vi "4-20mA Settings.vi"(8 "error in (no error)":errorcluster, 11 "PRM Config In":T1={"GUID"="", "Drop Coords"={"Horizontal"=0, "Vertical"=0}, "Process Name"="", "Settings"={"Cycle Period"=500.0, "PID 2 Parameters"={"Input Device"=enum."Default", "Output Device"=enum."Default", "Setpoint"=0.0, "PID gains"={"proportional gain (Kc)"=1.0, "integral time (Ti, min)"=0.01, "derivative time (Td, min)"=0.0}, "output range"={"output low"=0.02, "output high"=0.0}}, "Manual Entry"=0.0, "Auto?"=TRUE, "4-20mA Input Settings"={"Input Channel "=0}, "4-20mA Out Settings"={"Output DAQ Task"=""}, "Input Channel Tag Name "=""}, "Settings Load Count"=0} {"Settings"."PID 2 Parameters"."output range"."output low" format="%.2f"; "Settings"."PID 2 Parameters"."output range"."output high" min=0.0 max=100.0 format="%.2f"; "Settings"."PID 2 Parameters"."PID gains"."derivative time (Td, min)" format="%.3f"; "Settings"."PID 2 Parameters"."PID gains"."integral time (Ti, min)" format="%.3f"; "Settings"."PID 2 Parameters"."PID gains"."proportional gain (Kc)" format="%.3f"}) -> (0 "error out":errorcluster, 3 "PRM Config Out":T1={"GUID"="", "Drop Coords"={"Horizontal"=0, "Vertical"=0}, "Process Name"="", "Settings"={"Cycle Period"=500.0, "PID 2 Parameters"={"Input Device"=enum."Default", "Output Device"=enum."Default", "Setpoint"=0.0, "PID gains"={"proportional gain (Kc)"=1.0, "integral time (Ti, min)"=0.01, "derivative time (Td, min)"=0.0}, "output range"={"output low"=0.02, "output high"=0.0}}, "Manual Entry"=0.0, "Auto?"=TRUE, "4-20mA Input Settings"={"Input Channel "=0}, "4-20mA Out Settings"={"Output DAQ Task"=""}, "Input Channel Tag Name "=""}, "Settings Load Count"=0} {"Settings"."PID 2 Parameters"."output range"."output low" format="%.2f"; "Settings"."PID 2 Parameters"."output range"."output high" min=0.0 max=100.0 format="%.2f"; "Settings"."PID 2 Parameters"."PID gains"."derivative time (Td, min)" format="%.3f"; "Settings"."PID 2 Parameters"."PID gains"."integral time (Ti, min)" format="%.3f"; "Settings"."PID 2 Parameters"."PID gains"."proportional gain (Kc)" format="%.3f"})   [LabVIEW 2018, in "4-20mA Module.lvlib"]
uses:
  4-20mA Module.lvlib
  KNF Pump/Settings Cluster plus SIMDOS.ctl
  KNF Pump/KNF SIMDOS.lvlib
  Ismatec ISM 831C/Ismatec ISM 831C.lvlib
  VICI M50 Party Mode/VICI M6 M50 Party Mode.lvlib
  Masterflex 7550-30/Masterflex 7550-30.lvlib
  Mettler Toledo/Mettler Toledo.lvlib
  Bronkhorst M13 Flow Meter/Bronkhorst M13 Flow Meter.lvlib
  Bronkhorst M14 Flow Meter/Bronkhorst M14 Flow Meter.lvlib
  Settings/Settings.lvlib
  <vilib>/Utility/xml.llb/Write to XML File(string).vi
  <vilib>/Utility/miscctls.llb/LVPoint32TypeDef.ctl
  Masterflex 7550-30/Controls/Settings Cluster.ctl
  Mettler Toledo/Controls/Settings Cluster.ctl
  Bronkhorst M13 Flow Meter/Settings Cluster.ctl
  Measure Instrument/PID Input Enum.ctl
  Measure Instrument/PID 2 Output Enum.ctl
  Controls/Pressure Regulator COM Settings.ctl
  Pressure Transmitter/Pressure Transmitter Device Settings.ctl
  Pressure Transmitter/Pressure Transmitter Library.lvlib
  Controls/4-20mA Module Settings Cluster.ctl
  Controls/4-20mA Module Config Cluster.ctl
  Pressure Reg Module/Pressure Regulator Device Settings.ctl
  Pressure Reg Module/Pressure Regulator Library.lvlib
panel:
  out "Cancelled?":bool=TRUE
  in  "Cancel Button":bool
  in  "OK Button":bool
  in  "Settings Dialog":T12={"Cycle Period"=500.0, "Masterflex"={"VISA resource name"="", "Simulated?"=FALSE, "Pump Number"=1.0, "Reverse?"=FALSE}, "Mettler"={"VISA resource name"="", "Simulated?"=FALSE}, "Bronkhorst M13 Flow Meter"={"VISA resource name"="", "Simulated?"=FALSE}, "PID Parameters"={"Input Device"=enum."Default", "Output Device"=enum."Default", "PID gains"={"proportional gain (Kc)"=1.0, "integral time (Ti, min)"=0.01, "derivative time (Td, min)"=0.0}}, "PID Range"={"output high"=100.0, "output low"=0.0}, "Pressure Regulator Settings"={"Analog DAQ Task"="", "Digital DAQ Task"="", "Value"=0.02, "On?"=FALSE}} {"Pressure Regulator Settings"."Value" min=0.004 max=0.02; "PID Range"."output low" min=0.0 max=100.0 format="%.2f"; "PID Range"."output high" format="%.2f"; "PID Parameters"."PID gains"."derivative time (Td, min)" format="%.3f"; "PID Parameters"."PID gains"."integral time (Ti, min)" format="%.3f"; "PID Parameters"."PID gains"."proportional gain (Kc)" format="%.3f"; "Masterflex"."Pump Number" min=1.0 max=20.0 step=1.0}
  out "UI Refresh Needed?":bool
  # "Instrument Settings"
  # "Instrument Settings"
  # "Instrument Settings"
  # "Instrument Settings"
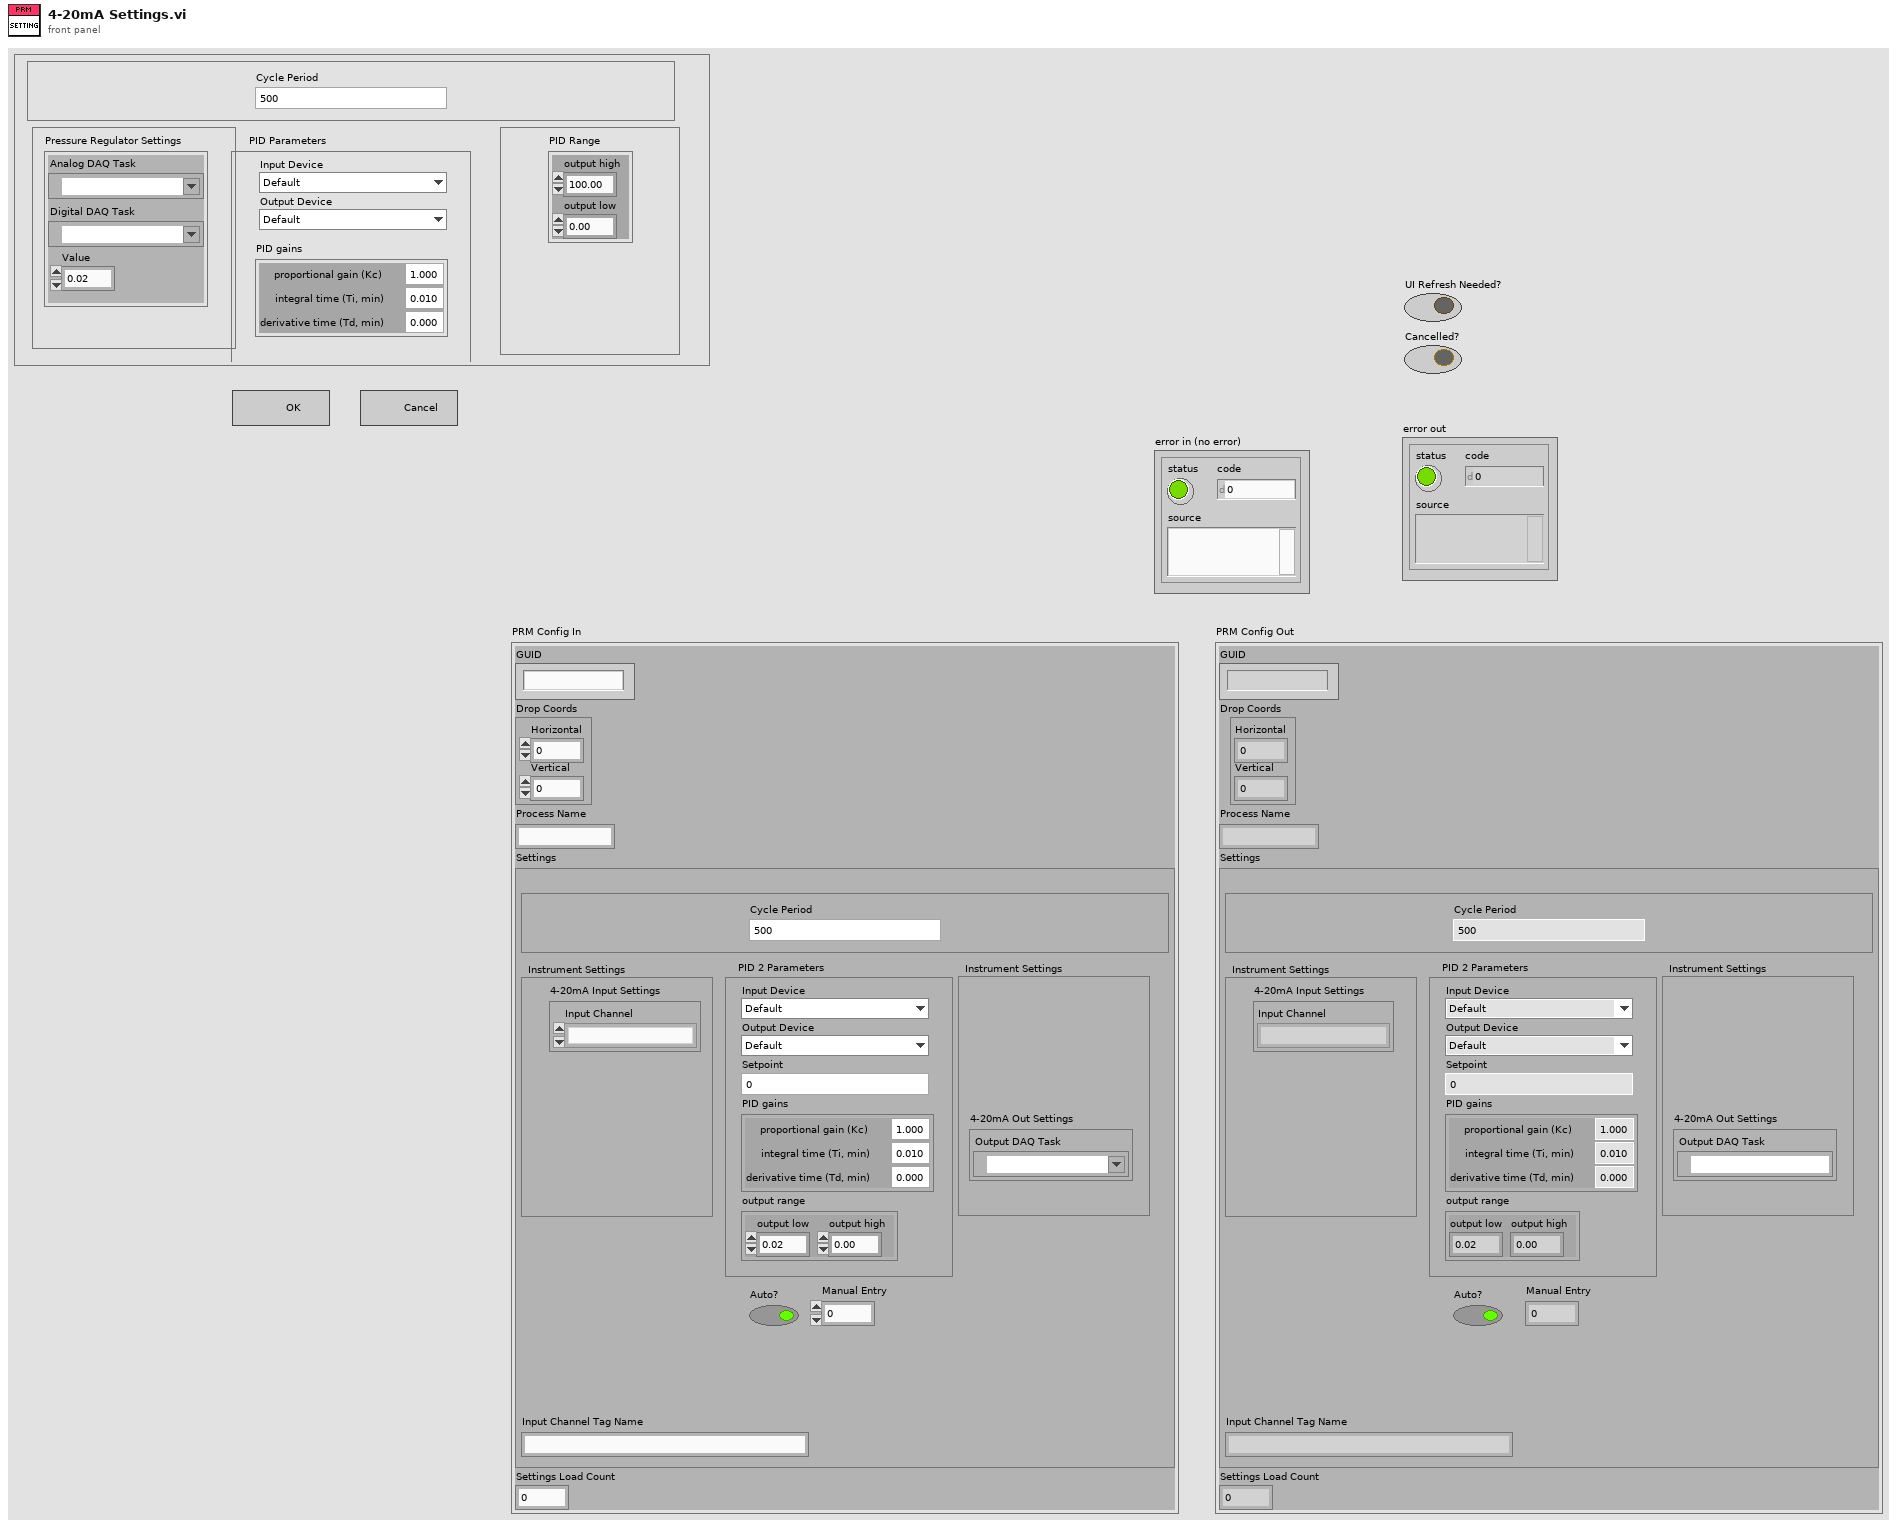
[diagram p1: front panel]
types:
  T1 = typedef "4-20mA Module.lvlib/4-20mA Module Config Cluster.ctl" = cluster{"GUID":string, "Drop Coords":T2, "Process Name":string, "Settings":T3, "Settings Load Count":i32}
  T2 = typedef "LVPoint32TypeDef.ctl" = cluster{"Horizontal":i32, "Vertical":i32}
  T3 = typedef "4-20mA Module.lvlib/4-20mA Module Settings Cluster.ctl" = cluster{"Cycle Period":dbl, "PID 2 Parameters":cluster{"Input Device":enum16{"Default", "4-20mA"}, "Output Device":enum16{"Default", "Equilibar Pressure Reg", "Flow Regulator"}, "Setpoint":dbl, "PID gains":cluster{"proportional gain (Kc)":dbl, "integral time (Ti, min)":dbl, "derivative time (Td, min)":dbl}, "output range":cluster{"output low":dbl, "output high":dbl}}, "Manual Entry":dbl, "Auto?":bool, "4-20mA Input Settings":T4, "4-20mA Out Settings":T5, "Input Channel Tag Name ":string}
  T4 = typedef "Pressure Transmitter Library.lvlib/Pressure Transmitter Device Settings.ctl" = cluster{"Input Channel ":u16}
  T5 = typedef "Pressure Regulator Library.lvlib/Pressure Regulator Device Settings.ctl" = cluster{"Output DAQ Task":refnum<k21>}
  T6 = typedef "Masterflex 7550-30.lvlib/Settings Cluster.ctl" = cluster{"VISA resource name":refnum<visa-resource-name>, "Simulated?":bool, "Pump Number":dbl, "Reverse?":bool}
  T7 = typedef "Mettler Toledo.lvlib/Settings Cluster.ctl" = cluster{"VISA resource name":refnum<visa-resource-name>, "Simulated?":bool}
  T8 = typedef "Bronkhorst M13 Flow Meter.lvlib/Settings Cluster.ctl" = cluster{"VISA resource name":refnum<visa-resource-name>, "Simulated?":bool}
  T9 = typedef "PID Input Enum.ctl" = enum16{"Default", "Bronkhorst M13", "Bronkhorst M14", "Scale Rate of Change"}
  T10 = typedef "PID 2 Output Enum.ctl" = enum16{"Default", "Ismatec ISM 831C", "Masterflex 7550-30", "VICI", "Tacmina QI", "KNF SIMDOS", "ASIA Type C", "FLOM UI-22-11", "SSI PR"}
  T11 = typedef "Pressure Regulator Module.lvlib/Pressure Regulator COM Settings.ctl" = cluster{"Analog DAQ Task":refnum<k21>, "Digital DAQ Task":refnum<k21>, "Value":dbl, "On?":bool}
  T12 = cluster{"Cycle Period":dbl, "Masterflex":T6, "Mettler":T7, "Bronkhorst M13 Flow Meter":T8, "PID Parameters":cluster{"Input Device":T9, "Output Device":T10, "PID gains":cluster{"proportional gain (Kc)":dbl, "integral time (Ti, min)":dbl, "derivative time (Td, min)":dbl}}, "PID Range":cluster{"output high":dbl, "output low":dbl}, "Pressure Regulator Settings":T11}
  T13 = typedef "KNF SIMDOS.lvlib/Settings Cluster plus SIMDOS.ctl" = cluster{"VISA resource name":refnum<visa-resource-name>, "Simulated?":bool}
  T14 = enum8{"Enabled", "Disabled", "Disabled and Grayed Out"}
  T15 = enum16{"Default", "Equilibar Pressure Reg", "Flow Regulator"}
  T16 = typedef "Ismatec ISM 831C.lvlib/Ismatech Settings Cluster.ctl" = cluster{"VISA resource name":refnum<visa-resource-name>, "Simulated?":bool, "Pump Number":dbl, "Reverse?":bool}
  T17 = cluster{"Input Device":T9, "Output Device":T10, "PID gains":cluster{"proportional gain (Kc)":dbl, "integral time (Ti, min)":dbl, "derivative time (Td, min)":dbl}}
  T18 = typedef "Bronkhorst M14 Flow Meter.lvlib/Settings Cluster.ctl" = cluster{"VISA resource name":refnum<visa-resource-name>, "Simulated?":bool}
  T19 = typedef "Tacmina QI.lvlib/Tacmina QI DAQ Setting.ctl" = cluster{"Analog DAQ Task":refnum<k21>, "Digital DAQ Task":refnum<k21>}
  T20 = typedef "ASIA Pump.lvlib/Pump Settings.ctl" = cluster{"ASIA Pump #":i32, "channel":i32, "Simulated":bool}
  T21 = typedef "VICI M50 Party Mode.lvlib/Settings Cluster.ctl" = cluster{"VISA resource name":refnum<visa-resource-name>, "Simulated?":bool, "Pump Letter":string, "Reverse?":bool}
  T22 = cluster{"proportional gain (Kc)":dbl, "integral time (Ti, min)":dbl, "derivative time (Td, min)":dbl}
  T23 = typedef "VICI M6 M50 Party Mode.lvlib/Settings Cluster.ctl" = cluster{"VISA resource name":refnum<visa-resource-name>, "Simulated?":bool, "Pump Letter":string, "Reverse?":bool}
  T24 = cluster{"Input Device":enum16{"Default", "4-20mA"}, "Output Device":enum16{"Default", "Equilibar Pressure Reg", "Flow Regulator"}, "Setpoint":dbl, "PID gains":cluster{"proportional gain (Kc)":dbl, "integral time (Ti, min)":dbl, "derivative time (Td, min)":dbl}, "output range":cluster{"output low":dbl, "output high":dbl}}
  T25 = cluster{"Output DAQ Task":refnum<k21>, void, void}
  T26 = cluster{"Cycle Period":dbl, "PID 2 Parameters":cluster{"Input Device":enum16{"Default", "4-20mA"}, "Output Device":enum16{"Default", "Equilibar Pressure Reg", "Flow Regulator"}, "Setpoint":dbl, "PID gains":cluster{"proportional gain (Kc)":dbl, "integral time (Ti, min)":dbl, "derivative time (Td, min)":dbl}, "output range":cluster{"output low":dbl, "output high":dbl}}, "Manual Entry":dbl, "Auto?":bool, "4-20mA Input Settings":T4, cluster{"Output DAQ Task":refnum<k21>, void, void}, void, void, void, void, void, void}
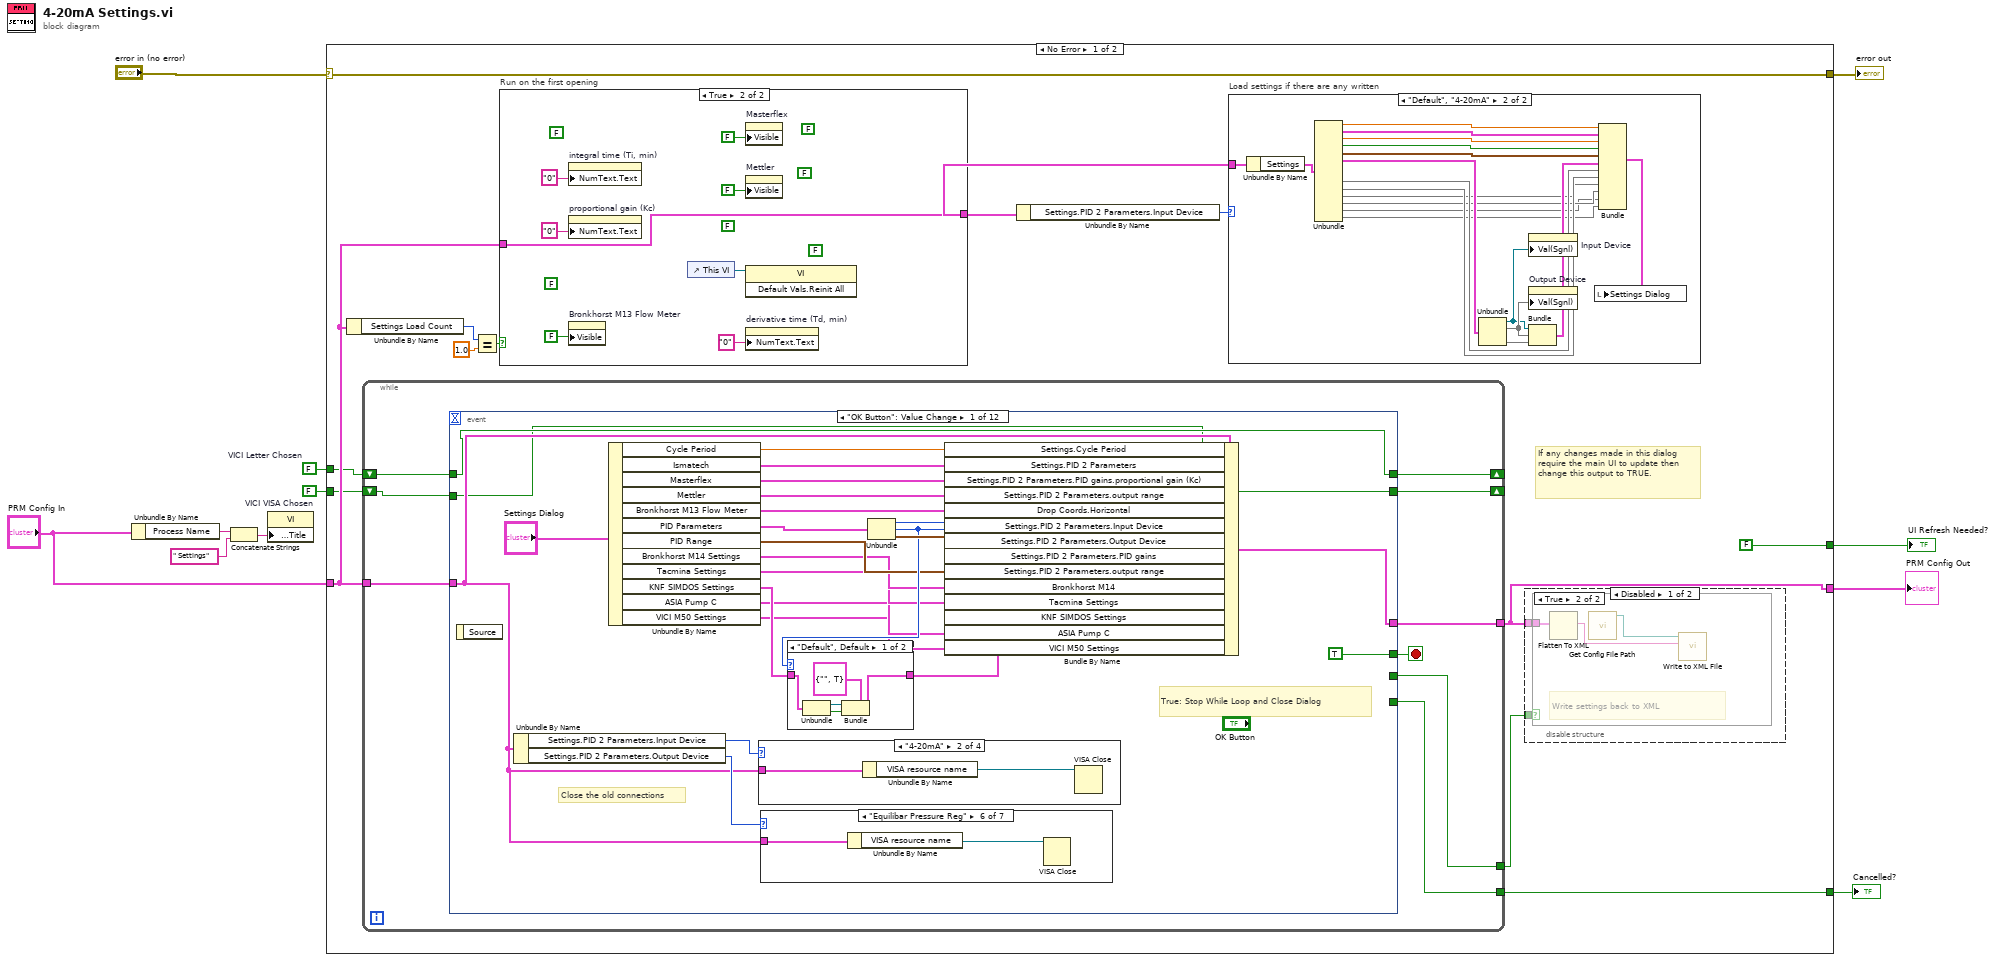
[diagram p0: block diagram]
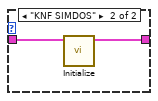
[diagram p6: hidden frame]
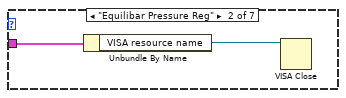
[diagram p8: hidden frame]
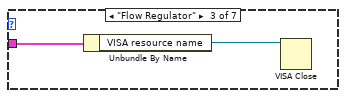
[diagram p9: hidden frame]
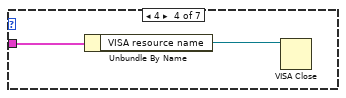
[diagram p10: hidden frame]
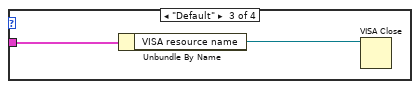
[diagram p14: hidden frame]
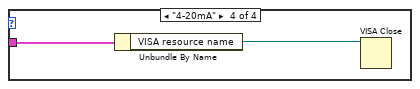
[diagram p15: hidden frame]
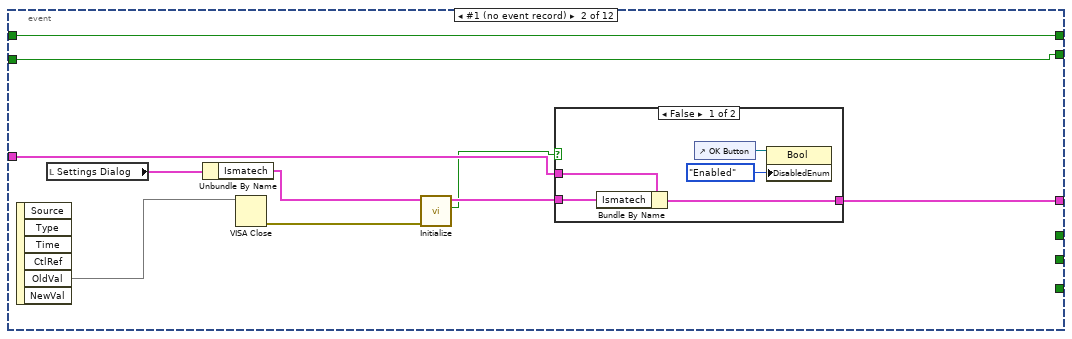
[diagram p16: hidden frame]
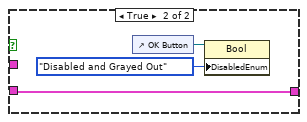
[diagram p17: hidden frame]
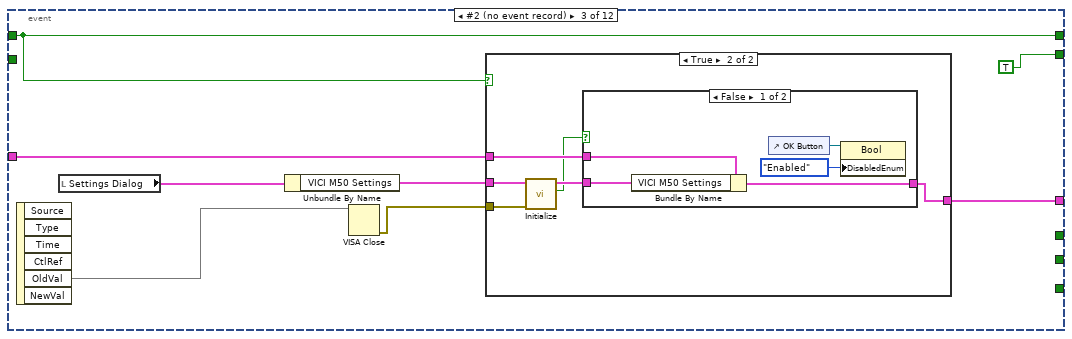
[diagram p18: hidden frame]
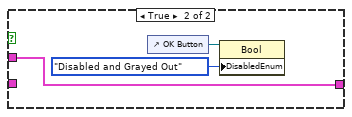
[diagram p20: hidden frame]
diagram:
  w3 = FALSE  # VICI VISA Chosen
  w4 = FALSE  # VICI Letter Chosen
  n1 = Unbundle By Name("PRM Config In") -> ("Process Name"=w7:string)
  n2 = Concatenate Strings(w7, " Settings" ("string")) -> (w6:string)
  n3 = property class="VI"("Front Panel.Title"=w6) -> ()  [unwired: 2 in, 2 out]
  n4 = case shown="No Error" "error in (no error)" {
    selector: "error in (no error)" -> [w24 w372]
    tunnel: [w24 w372] -> w11
    tunnel: "PRM Config In" -> [w20 w371]
    tunnel: [w22 w371] -> w1
    tunnel: [FALSE ("UI Refresh Needed?") _] -> w10
    tunnel: [w21 TRUE ("UI Refresh Needed?")] -> w9
    tunnel: w4 -> [w13 _]
    tunnel: w3 -> [w12 _]
    frame No Error {
      # "If any changes made in this dialog require the main UI to update then change this output to TRUE."
      n5 = Unbundle By Name(w20) -> ("Settings Load Count"=w19:i32)
      n6 = while {
        tunnel: [w71] -> w17
        tunnel: [w70] -> w22
        tunnel: w20 -> [w69]
        tunnel: [w67] -> w21
        shift-right: [w66] -> _
        shift-left: w13 -> [w65]
        shift-right: [w64] -> _
        shift-left: w12 -> [w63]
        stop <- w68 stop-if-true
        n7 = event shown="[0] \"OK Button\": Value Change" {
          selector: _ -> [_ _ _ _ _ _ _ _ _ _ _ _]
          dyn-events: _ -> [_ _ _ _ _ _ _ _ _ _ _ _]
          timeout: _ -> [_ _ _ _ _ _ _ _ _ _ _ _]
          tunnel: [w95 w127 w144 w165 w185 w205 w223 w240 w258 w272 w313 w369] -> w70
          tunnel: w69 -> [w82 w126 w143 w164 w186 w206 w224 w239 w257 w271 w313 w369]
          tunnel: [FALSE ("UI Refresh Needed?") _ _ _ _ _ _ _ _ _ _ FALSE ("UI Refresh Needed?")] -> w71
          tunnel: [TRUE _ _ _ _ _ _ _ _ _ _ TRUE] -> w68
          tunnel: [FALSE ("UI Refresh Needed?") _ _ _ _ _ _ _ _ _ _ TRUE ("UI Refresh Needed?")] -> w67
          tunnel: [w73 w120 w137 TRUE w181 w199 w217 w235 w253 w270 w312 w365] -> w66
          tunnel: w65 -> [w73 w120 w137 _ w181 w199 w217 w235 w253 w270 w312 w365]
          tunnel: [w72 w119 TRUE w160 w180 w198 w216 w234 w252 w269 w311 w364] -> w64
          tunnel: w63 -> [w72 w119 _ w160 w180 w198 w216 w234 w252 w269 w311 w364]
          event "OK Button": Value Change {
            # "Close the old connections"
            # "True: Stop While Loop and Close Dialog"
            n8 = event-data() -> ()  [unwired: 1 in, 1 out]
            n9 = Unbundle By Name(w82) -> ("Settings.PID 2 Parameters.Input Device"=w84:enum16{"Default", "4-20mA"}, "Settings.PID 2 Parameters.Output Device"=w83:T15)
            n10 = Unbundle By Name("Settings Dialog") -> ("Cycle Period"=w93:dbl, "Ismatech"=w92:T16, "Masterflex"=w91:T6, "Mettler"=w90:T7, "Bronkhorst M13 Flow Meter"=w89:T8, "PID Parameters"=w88:T17, "PID Range"=w80:cluster{"output high":dbl, "output low":dbl}, "Bronkhorst M14 Settings"=w79:T18, "Tacmina Settings"=w78:T19, "KNF SIMDOS Settings"=w76:T13, "ASIA Pump C"=w75:T20, "VICI M50 Settings"=w74:T21)
            n11 = case shown="\"4-20mA\"" w84 {
              tunnel: w82 -> [_ w114 w115 w117]
              frame "Default", Default {
              }
              frame "4-20mA" {
                n12 = Unbundle By Name(w114) -> ("VISA resource name"=w113:refnum<visa-resource-name>)
                n13 = VISA Close(VISA resource name=w113) -> ()  [unwired: 1 in, 1 out]
              }
              frame "Default" {
                n14 = Unbundle By Name(w115) -> ("VISA resource name"=w116:refnum<visa-resource-name>)
                n15 = VISA Close(VISA resource name=w116) -> ()  [unwired: 1 in, 1 out]
              }
              frame "4-20mA" {
                n16 = Unbundle By Name(w117) -> ("VISA resource name"=w118:refnum<visa-resource-name>)
                n17 = VISA Close(VISA resource name=w118) -> ()  [unwired: 1 in, 1 out]
              }
            }
            n18 = case shown="\"KNF SIMDOS\"" w83 {
              tunnel: w82 -> [_ w105 w107 w109 _ w112 _]
              frame "Default", Default {
              }
              frame "Equilibar Pressure Reg" {
                n19 = Unbundle By Name(w105) -> ("VISA resource name"=w106:refnum<visa-resource-name>)
                n20 = VISA Close(VISA resource name=w106) -> ()  [unwired: 1 in, 1 out]
              }
              frame "Flow Regulator" {
                n21 = Unbundle By Name(w107) -> ("VISA resource name"=w108:refnum<visa-resource-name>)
                n22 = VISA Close(VISA resource name=w108) -> ()  [unwired: 1 in, 1 out]
              }
              frame 4 {
                n23 = Unbundle By Name(w109) -> ("VISA resource name"=w110:refnum<visa-resource-name>)
                n24 = VISA Close(VISA resource name=w110) -> ()  [unwired: 1 in, 1 out]
              }
              frame 3 {
                # "No VISA to Close"
              }
              frame "Equilibar Pressure Reg" {
                n25 = Unbundle By Name(w112) -> ("VISA resource name"=w111:refnum<visa-resource-name>)
                n26 = VISA Close(VISA resource name=w111) -> ()  [unwired: 1 in, 1 out]
              }
              frame "Default" {
                # "No VISA to Close"
              }
            }
            n27 = Unbundle(w88) -> ("Input Device"=w86:T9, "Output Device"=w81:T10, "PID gains"=w87:T22)
            n28 = case shown="\"Default\", Default" w81 {
              tunnel: w76 -> [w102 w103]
              tunnel: [w101 w104] -> w77
              frame "Default", Default {
                n29 = Unbundle(w102) -> ("VISA resource name"=w99:refnum<visa-resource-name>, "Simulated?"=w98:bool)
                n30 = Bundle(cluster=T13 {"VISA resource name"="", "Simulated?"=TRUE} ("KNF Settings"), "VISA resource name"=w99, "Simulated?"=w98) -> (w101:T13)
              }
              frame "KNF SIMDOS" {
                n31 = call "Initialize.vi"("KNF Settings"=w103) -> ("KNF Settings"=w104:T13)  [unwired: 7 in, 3 out]
              }
            }
            n32 = Bundle By Name(cluster=w82, "Settings.Cycle Period"=w93, "Settings.PID 2 Parameters"=w92, "Settings.PID 2 Parameters.PID gains.proportional gain (Kc)"=w91, "Settings.PID 2 Parameters.output range"=w90, "Drop Coords.Horizontal"=w89, "Settings.PID 2 Parameters.Input Device"=w86, "Settings.PID 2 Parameters.Output Device"=w81, "Settings.PID 2 Parameters.PID gains"=w87, "Settings.PID 2 Parameters.output range"=w80, "Bronkhorst M14"=w79, "Tacmina Settings"=w78, "KNF SIMDOS Settings"=w77, "ASIA Pump C"=w75, "VICI M50 Settings"=w74) -> (w95:T1)
          }
          event #1 (no event record) {
            n33 = event-data() -> ("OldVal"=w122)  [unwired: 1 in, 5 out]
            n34 = local read "Settings Dialog"() -> (w125:T12)
            n35 = Unbundle By Name(w125) -> ("Ismatech"=w124:T16)
            n36 = VISA Close(VISA resource name=w122) -> (error out=w123:errorcluster)  [unwired: 1 in]
            n37 = call "Initialize.vi"("error in (no error)"=w123, "Ismatech Settings"=w124) -> ("No Pump Connected"=w121:bool, "Ismatech Settings"=w128:T16)  [unwired: 6 in, 2 out]
            n38 = case shown="False" w121 {
              tunnel: w128 -> [w133 _]
              tunnel: [w132 w136] -> w127
              tunnel: w126 -> [w131 w136]
              frame False {
                n39 = Bundle By Name(cluster=w131, "Ismatech"=w133) -> (w132:T1)
                n40 = control-ref of="OK Button"() -> (w129:refnum<vi>)
                n41 = property on="Property Node" class="Bool"(reference=w129, "DisabledEnum"=T14."Enabled" ("Disabled")) -> ()  [unwired: 1 in, 2 out]
              }
              frame True {
                n42 = control-ref of="OK Button"() -> (w134:refnum<vi>)
                n43 = property on="Property Node" class="Bool"(reference=w134, "DisabledEnum"=T14."Disabled and Grayed Out" ("Disabled")) -> ()  [unwired: 1 in, 2 out]
              }
            }
          }
          event #2 (no event record) {
            n44 = event-data() -> ("OldVal"=w139)  [unwired: 1 in, 5 out]
            n45 = local read "Settings Dialog"() -> (w142:T12)
            n46 = Unbundle By Name(w142) -> ("VICI M50 Settings"=w141:T21)
            n47 = VISA Close(VISA resource name=w139) -> (error out=w140:errorcluster)  [unwired: 1 in]
            n48 = case shown="True" w137 {
              tunnel: [w145 w151] -> w144
              tunnel: w143 -> [w145 w150]
              tunnel: w141 -> [_ w148]
              tunnel: w140 -> [_ w147]
              frame False {
              }
              frame True {
                n49 = call "Initialize.vi"("error in (no error)"=w147, "VICI Settings"=w148) -> ("No Pump Connected"=w146:bool, "VICI Settings"=w149:T23)  [unwired: 6 in, 2 out]
                n50 = case shown="False" w146 {
                  tunnel: [w156 w159] -> w151
                  tunnel: w150 -> [w155 w159]
                  tunnel: w149 -> [w152 _]
                  frame False {
                    n51 = Bundle By Name(cluster=w155, "VICI M50 Settings"=w152) -> (w156:T1)
                    n52 = control-ref of="OK Button"() -> (w153:refnum<vi>)
                    n53 = property on="Property Node" class="Bool"(reference=w153, "DisabledEnum"=T14."Enabled" ("Disabled")) -> ()  [unwired: 1 in, 2 out]
                  }
                  frame True {
                    n54 = control-ref of="OK Button"() -> (w157:refnum<vi>)
                    n55 = property on="Property Node" class="Bool"(reference=w157, "DisabledEnum"=T14."Disabled and Grayed Out" ("Disabled")) -> ()  [unwired: 1 in, 2 out]
                  }
                }
              }
            }
          }
          event #3 (no event record) {
            n56 = event-data() -> ()  [unwired: 1 in, 1 out]
            n57 = local read "Settings Dialog"() -> (w163:T12)
            n58 = Unbundle By Name(w163) -> ("VICI M50 Settings"=w162:T21)
            n59 = case shown="True" w160 {
              tunnel: [w166 w171] -> w165
              tunnel: w164 -> [w166 w170]
              tunnel: w162 -> [_ w168]
              frame False {
              }
              frame True {
                n60 = call "Initialize.vi"("VICI Settings"=w168) -> ("No Pump Connected"=w167:bool, "VICI Settings"=w169:T23)  [unwired: 7 in, 2 out]
                n61 = case shown="False" w167 {
                  tunnel: [w176 w179] -> w171
                  tunnel: w170 -> [w175 w179]
                  tunnel: w169 -> [w172 _]
                  frame False {
                    n62 = Bundle By Name(cluster=w175, "VICI M50 Settings"=w172) -> (w176:T1)
                    n63 = control-ref of="OK Button"() -> (w173:refnum<vi>)
                    n64 = property on="Property Node" class="Bool"(reference=w173, "DisabledEnum"=T14."Enabled" ("Disabled")) -> ()  [unwired: 1 in, 2 out]
                  }
                  frame True {
                    n65 = control-ref of="OK Button"() -> (w177:refnum<vi>)
                    n66 = property on="Property Node" class="Bool"(reference=w177, "DisabledEnum"=T14."Disabled and Grayed Out" ("Disabled")) -> ()  [unwired: 1 in, 2 out]
                  }
                }
              }
            }
          }
          event Value Change {
            n67 = event-data() -> ("OldVal"=w183:refnum<visa-resource-name>)  [unwired: 1 in, 5 out]
            n68 = local read "Settings Dialog"() -> (w187:T12)
            n69 = Unbundle By Name(w187) -> ("Masterflex"=w189:T6)
            n70 = VISA Close(VISA resource name=w183) -> (error out=w184:errorcluster)  [unwired: 1 in]
            n71 = call "Initialize.vi"("error in (no error)"=w184, "Masterflex Settings in"=w189) -> ("No Pump Connected"=w182:bool, "Masterflex Settings out"=w188:T6)  [unwired: 6 in, 2 out]
            n72 = case shown="False" w182 {
              tunnel: w188 -> [w190 _]
              tunnel: w186 -> [w194 w197]
              tunnel: [w193 w197] -> w185
              frame False {
                n73 = Bundle By Name(cluster=w194, "Masterflex"=w190) -> (w193:T1)
                n74 = control-ref of="OK Button"() -> (w191:refnum<vi>)
                n75 = property on="Property Node" class="Bool"(reference=w191, "DisabledEnum"=T14."Enabled" ("Disabled")) -> ()  [unwired: 1 in, 2 out]
              }
              frame True {
                n76 = control-ref of="OK Button"() -> (w195:refnum<vi>)
                n77 = property on="Property Node" class="Bool"(reference=w195, "DisabledEnum"=T14."Disabled and Grayed Out" ("Disabled")) -> ()  [unwired: 1 in, 2 out]
              }
            }
          }
          event #5 (no event record) {
            n78 = event-data() -> ("OldVal"=w204)  [unwired: 1 in, 5 out]
            n79 = local read "Settings Dialog"() -> (w207:T12)
            n80 = Unbundle By Name(w207) -> ("KNF SIMDOS Settings"=w202:T13)
            n81 = VISA Close(VISA resource name=w204) -> (error out=w203:errorcluster)  [unwired: 1 in]
            n82 = call "Initialize.vi"("error in (no error)"=w203, "KNF Settings"=w202) -> ("No Pump Connected"=w200:bool, "KNF Settings"=w201:T13)  [unwired: 6 in, 2 out]
            n83 = case shown="False" w200 {
              tunnel: w206 -> [w212 w215]
              tunnel: [w211 w215] -> w205
              tunnel: w201 -> [w210 _]
              frame False {
                n84 = Bundle By Name(cluster=w212, "KNF SIMDOS Settings"=w210) -> (w211:T1)
                n85 = control-ref of="OK Button"() -> (w208:refnum<vi>)
                n86 = property on="Property Node" class="Bool"(reference=w208, "DisabledEnum"=T14."Enabled" ("Disabled")) -> ()  [unwired: 1 in, 2 out]
              }
              frame True {
                n87 = control-ref of="OK Button"() -> (w213:refnum<vi>)
                n88 = property on="Property Node" class="Bool"(reference=w213, "DisabledEnum"=T14."Disabled and Grayed Out" ("Disabled")) -> ()  [unwired: 1 in, 2 out]
              }
            }
          }
          event Value Change {
            n89 = event-data() -> ("OldVal"=w220:refnum<visa-resource-name>)  [unwired: 1 in, 5 out]
            n90 = local read "Settings Dialog"() -> (w225:T12)
            n91 = Unbundle By Name(w225) -> ("Mettler"=w222:T7)
            n92 = VISA Close(VISA resource name=w220) -> (error out=w219:errorcluster)  [unwired: 1 in]
            n93 = call "Initialize.vi"("error in (no error)"=w219, "Mettler Settings in"=w222) -> ("No Scale Connected"=w218:bool, "Mettler Settings out"=w221:T7)  [unwired: 7 in, 1 out]
            n94 = case shown="False" w218 {
              tunnel: w224 -> [w230 w233]
              tunnel: [w229 w233] -> w223
              tunnel: w221 -> [w228 _]
              frame False {
                n95 = Bundle By Name(cluster=w230, "Mettler"=w228) -> (w229:T1)
                n96 = control-ref of="OK Button"() -> (w226:refnum<vi>)
                n97 = property on="Property Node" class="Bool"(reference=w226, "DisabledEnum"=T14."Enabled" ("Disabled")) -> ()  [unwired: 1 in, 2 out]
              }
              frame True {
                n98 = control-ref of="OK Button"() -> (w231:refnum<vi>)
                n99 = property on="Property Node" class="Bool"(reference=w231, "DisabledEnum"=T14."Disabled and Grayed Out" ("Disabled")) -> ()  [unwired: 1 in, 2 out]
              }
            }
          }
          event Value Change {
            n100 = event-data() -> ("OldVal"=w237:refnum<visa-resource-name>)  [unwired: 1 in, 5 out]
            n101 = local read "Settings Dialog"() -> (w243:T12)
            n102 = Unbundle By Name(w243) -> ("Bronkhorst M13 Flow Meter"=w242:T8)
            n103 = VISA Close(VISA resource name=w237) -> (error out=w238:errorcluster)  [unwired: 1 in]
            n104 = call "Initialize.vi"("error in (no error)"=w238, "Bronkhorst Settings in"=w242) -> ("No Meter Connnected"=w236:bool, "Bronkhorst Settings out"=w241:T8)  [unwired: 7 in, 1 out]
            n105 = case shown="False" w236 {
              tunnel: w241 -> [w248 _]
              tunnel: [w247 w251] -> w240
              tunnel: w239 -> [w246 w251]
              frame False {
                n106 = Bundle By Name(cluster=w246, "Bronkhorst M13 Flow Meter"=w248) -> (w247:T1)
                n107 = control-ref of="OK Button"() -> (w244:refnum<vi>)
                n108 = property on="Property Node" class="Bool"(reference=w244, "DisabledEnum"=T14."Enabled" ("Disabled")) -> ()  [unwired: 1 in, 2 out]
              }
              frame True {
                n109 = control-ref of="OK Button"() -> (w249:refnum<vi>)
                n110 = property on="Property Node" class="Bool"(reference=w249, "DisabledEnum"=T14."Disabled and Grayed Out" ("Disabled")) -> ()  [unwired: 1 in, 2 out]
              }
            }
          }
          event #8 (no event record) {
            n111 = event-data() -> ("OldVal"=w255)  [unwired: 1 in, 5 out]
            n112 = local read "Settings Dialog"() -> (w261:T12)
            n113 = Unbundle By Name(w261) -> ("Bronkhorst M14 Settings"=w260:T18)
            n114 = VISA Close(VISA resource name=w255) -> (error out=w256:errorcluster)  [unwired: 1 in]
            n115 = call "Initialize.vi"("error in (no error)"=w256, "Bronkhorst Settings in"=w260) -> ("No Meter Connected"=w254:bool, "Bronkhorst Settings out"=w259:T18)  [unwired: 7 in, 1 out]
            n116 = case shown="False" w254 {
              tunnel: w259 -> [w266 _]
              tunnel: [w265 w268] -> w258
              tunnel: w257 -> [w264 w268]
              frame False {
                n117 = Bundle By Name(cluster=w264, "Bronkhorst M14"=w266) -> (w265:T1)
                n118 = control-ref of="OK Button"() -> (w262:refnum<vi>)
                n119 = property on="Property Node" class="Bool"(reference=w262, "DisabledEnum"=T14."Enabled" ("Disabled")) -> ()  [unwired: 1 in, 2 out]
              }
              frame True {
                n120 = property on="OK Button" class="Bool"("DisabledEnum"=T14."Disabled and Grayed Out" ("Disabled")) -> ()  [unwired: 2 in, 2 out]
              }
            }
          }
          event Value Change {
            n121 = event-data() -> ("NewVal"=w273:T9)  [unwired: 1 in, 5 out]
            n122 = case "Show the correct settings" shown="\"Bronkhorst M13\"" w273 {
              tunnel: [w274 w284 w294 w305] -> w272
              tunnel: w271 -> [w274 w284 w294 w305]
              frame "Bronkhorst M13" {
                w275 = FALSE ("Visible")
                n123 = Unbundle By Name(w274) -> ("Settings.PID 2 Parameters.Input Device"=w276:enum16{"Default", "4-20mA"})
                n124 = property on="Mettler" class="Clust (strict)"("Visible"=FALSE) -> ()  [unwired: 2 in, 2 out]
                n125 = property on="Bronkhorst M13 Flow Meter" class="Clust (strict)"("Visible"=TRUE) -> ()  [unwired: 2 in, 2 out]
                n126 = Unbundle By Name(w274) -> ("VISA resource name"=w277:refnum<visa-resource-name>)
                n127 = case shown="\"Default\", Default" w276 {
                  frame "Default", Default {
                    n128 = property on="derivative time (Td, min)" class="DigNum (strict)"("NumText.Text"="0" ("Numeric Text.Text")) -> ()  [unwired: 2 in, 2 out]
                    n129 = property on="proportional gain (Kc)" class="DigNum (strict)"("NumText.Text"=".4" ("Numeric Text.Text")) -> ()  [unwired: 2 in, 2 out]
                    n130 = property on="integral time (Ti, min)" class="DigNum (strict)"("NumText.Text"="0.035" ("Numeric Text.Text")) -> ()  [unwired: 2 in, 2 out]
                  }
                  frame "Default", "4-20mA" {
                  }
                }
                n131 = control-ref of="VISA resource name"() -> (w278:refnum<vi>)
                n132 = property on="Property Node" class="VISAName"(reference=w278, "Value"=w277) -> ()  [unwired: 1 in, 2 out]
              }
              frame "Bronkhorst M14" {
                w285 = TRUE ("Visible")
                n133 = Unbundle By Name(w284) -> ("Settings.PID 2 Parameters.Input Device"=w286:enum16{"Default", "4-20mA"})
                n134 = property on="Mettler" class="Clust (strict)"("Visible"=FALSE) -> ()  [unwired: 2 in, 2 out]
                n135 = property on="Bronkhorst M13 Flow Meter" class="Clust (strict)"("Visible"=FALSE) -> ()  [unwired: 2 in, 2 out]
                n136 = Unbundle By Name(w284) -> ("VISA resource name"=w287:refnum<visa-resource-name>)
                n137 = control-ref of="VISA resource name"() -> (w288:refnum<vi>)
                n138 = case shown="\"Default\", Default" w286 {
                  frame "Default", Default {
                    n139 = property on="derivative time (Td, min)" class="DigNum (strict)"("NumText.Text"="0" ("Numeric Text.Text")) -> ()  [unwired: 2 in, 2 out]
                    n140 = property on="proportional gain (Kc)" class="DigNum (strict)"("NumText.Text"=".4" ("Numeric Text.Text")) -> ()  [unwired: 2 in, 2 out]
                    n141 = property on="integral time (Ti, min)" class="DigNum (strict)"("NumText.Text"="0.035" ("Numeric Text.Text")) -> ()  [unwired: 2 in, 2 out]
                  }
                  frame "Default", "4-20mA" {
                  }
                }
                n142 = property on="Property Node" class="VISAName"(reference=w288, "Value"=w287) -> ()  [unwired: 1 in, 2 out]
              }
              frame "Scale Rate of Change" {
                w295 = FALSE ("Visible")
                n143 = Unbundle By Name(w294) -> ("Settings.PID 2 Parameters.Input Device"=w296:enum16{"Default", "4-20mA"})
                n144 = property on="Mettler" class="Clust (strict)"("Visible"=TRUE) -> ()  [unwired: 2 in, 2 out]
                n145 = property on="Bronkhorst M13 Flow Meter" class="Clust (strict)"("Visible"=FALSE) -> ()  [unwired: 2 in, 2 out]
                n146 = Unbundle By Name(w294) -> ("VISA resource name"=w298:refnum<visa-resource-name>)
                n147 = control-ref of="VISA resource name"() -> (w297:refnum<vi>)
                n148 = case shown="\"Default\", Default" w296 {
                  frame "Default", Default {
                    n149 = property on="derivative time (Td, min)" class="DigNum (strict)"("NumText.Text"="0" ("Numeric Text.Text")) -> ()  [unwired: 2 in, 2 out]
                    n150 = property on="proportional gain (Kc)" class="DigNum (strict)"("NumText.Text"=".4" ("Numeric Text.Text")) -> ()  [unwired: 2 in, 2 out]
                    n151 = property on="integral time (Ti, min)" class="DigNum (strict)"("NumText.Text"="0.035" ("Numeric Text.Text")) -> ()  [unwired: 2 in, 2 out]
                  }
                  frame "Default", "4-20mA" {
                  }
                }
                n152 = property on="Property Node" class="VISAName"(reference=w297, "Value"=w298) -> ()  [unwired: 1 in, 2 out]
              }
              frame "Default", Default {
                w304 = FALSE ("Visible")
                n153 = property on="Bronkhorst M13 Flow Meter" class="Clust (strict)"("Visible"=FALSE) -> ()  [unwired: 2 in, 2 out]
                n154 = property on="Mettler" class="Clust (strict)"("Visible"=FALSE) -> ()  [unwired: 2 in, 2 out]
                n155 = property on="proportional gain (Kc)" class="DigNum (strict)"("NumText.Text"="0" ("Numeric Text.Text")) -> ()  [unwired: 2 in, 2 out]
                n156 = property on="integral time (Ti, min)" class="DigNum (strict)"("NumText.Text"="0" ("Numeric Text.Text")) -> ()  [unwired: 2 in, 2 out]
                n157 = property on="derivative time (Td, min)" class="DigNum (strict)"("NumText.Text"="0" ("Numeric Text.Text")) -> ()  [unwired: 2 in, 2 out]
              }
            }
          }
          event Value Change {
            n158 = event-data() -> ("NewVal"=w314:T10)  [unwired: 1 in, 5 out]
            n159 = case "Show the correct settings" shown="\"VICI\"" w314 {
              tunnel: w313 -> [w318 w326 w335 _ _ w350 w355]
              frame "Ismatec ISM 831C" {
                w316 = FALSE ("Visible")
                (unwired) FALSE ("Visible")
                w317 = FALSE ("Visible")
                w315 = FALSE ("Visible")
                w322 = TRUE ("Visible")
                n160 = Unbundle By Name(w318) -> ("VISA resource name"=w319:refnum<visa-resource-name>)
                n161 = property on="Masterflex" class="Clust (strict)"("Visible"=FALSE) -> ()  [unwired: 2 in, 2 out]
                n162 = property on="Property Node" class="VISAName"("Value"=w319) -> (reference=w320:refnum<vi>)  [unwired: 1 in, 2 out]
              }
              frame "Masterflex 7550-30" {
                w323 = FALSE ("Visible")
                w324 = FALSE ("Visible")
                w325 = FALSE ("Visible")
                (unwired) FALSE ("Visible")
                w330 = FALSE ("Visible")
                n163 = property on="Masterflex" class="Clust (strict)"("Visible"=TRUE) -> ()  [unwired: 2 in, 2 out]
                n164 = Unbundle By Name(w326) -> ("VISA resource name"=w327:refnum<visa-resource-name>)
                n165 = control-ref of="VISA resource name"() -> (w328:refnum<vi>)
                n166 = property on="Property Node" class="VISAName"(reference=w328, "Value"=w327) -> ()  [unwired: 1 in, 2 out]
              }
              frame "VICI" {
                w331 = FALSE ("Visible")
                w332 = FALSE ("Visible")
                w333 = FALSE ("Visible")
                (unwired) TRUE ("Visible")
                w336 = FALSE ("Visible")
                n167 = property on="Masterflex" class="Clust (strict)"("Visible"=FALSE) -> ()  [unwired: 2 in, 2 out]
                n168 = Unbundle By Name(w335) -> ("VISA resource name"=w334:refnum<visa-resource-name>)
              }
              frame "Default", Default {
                w339 = FALSE ("Visible")
                w340 = FALSE ("Visible")
                w341 = FALSE ("Visible")
                w343 = FALSE ("Visible")
                w338 = FALSE ("Visible")
                n169 = property on="Masterflex" class="Clust (strict)"("Visible"=FALSE) -> ()  [unwired: 2 in, 2 out]
              }
              frame "Tacmina QI" {
                w344 = FALSE ("Visible")
                w345 = FALSE ("Visible")
                w346 = TRUE ("Visible")
                (unwired) FALSE ("Visible")
                w347 = FALSE ("Visible")
                n170 = property on="Masterflex" class="Clust (strict)"("Visible"=FALSE) -> ()  [unwired: 2 in, 2 out]
              }
              frame "KNF SIMDOS" {
                w349 = FALSE ("Visible")
                (unwired) TRUE ("Visible")
                w352 = FALSE ("Visible")
                (unwired) FALSE ("Visible")
                w353 = FALSE ("Visible")
                n171 = property on="Masterflex" class="Clust (strict)"("Visible"=FALSE) -> ()  [unwired: 2 in, 2 out]
                n172 = Unbundle By Name(w350) -> ("VISA resource name"=w351:refnum<visa-resource-name>)
              }
              frame "ASIA Type C" {
                w360 = TRUE ("Visible")
                (unwired) FALSE ("Visible")
                w361 = FALSE ("Visible")
                (unwired) FALSE ("Visible")
                w363 = FALSE ("Visible")
                n173 = Unbundle By Name(w355) -> ("ASIA Pump #"=w358:i32)
                n174 = Unbundle By Name(w355) -> ("channel"=w357:i32)
                n175 = property on="Masterflex" class="Clust (strict)"("Visible"=FALSE) -> ()  [unwired: 2 in, 2 out]
                n176 = property on="Property Node" class="DigNum (strict)"("Value"=w358) -> (reference=w359:refnum<vi>)  [unwired: 1 in, 2 out]
                n177 = property on="Property Node" class="DigNum (strict)"("Value"=w357) -> (reference=w356:refnum<vi>)  [unwired: 1 in, 2 out]
              }
            }
          }
          event "Cancel Button": Value Change; Panel Close {
            # "True: Stop While Loop and Close Dialog"
            n178 = event-data() -> ()  [unwired: 1 in, 1 out]
          }
        }
      }
      n179 = Equal?(x=w19, y=1.0) -> (x = y?=w16:bool)
      n180 = case "Run on the first opening" shown="True" w16 {
        tunnel: w20 -> [w49 w55]
        tunnel: [w49 w55] -> w14
        frame False {
        }
        frame True {
          w51 = FALSE ("Visible")
          w52 = FALSE ("Visible")
          w53 = FALSE ("Visible")
          w54 = FALSE ("Visible")
          (unwired) FALSE ("Visible")
          w50 = FALSE ("Visible")
          n181 = property on="integral time (Ti, min)" class="DigNum (strict)"("NumText.Text"="0" ("Numeric Text.Text")) -> ()  [unwired: 2 in, 2 out]
          n182 = property on="proportional gain (Kc)" class="DigNum (strict)"("NumText.Text"="0" ("Numeric Text.Text")) -> ()  [unwired: 2 in, 2 out]
          n183 = property on="Bronkhorst M13 Flow Meter" class="Clust (strict)"("Visible"=FALSE) -> ()  [unwired: 2 in, 2 out]
          n184 = control-ref of="This VI"() -> (w56:refnum<vi>)
          n185 = property on="Masterflex" class="Clust (strict)"("Visible"=FALSE) -> ()  [unwired: 2 in, 2 out]
          n186 = property on="Mettler" class="Clust (strict)"("Visible"=FALSE) -> ()  [unwired: 2 in, 2 out]
          n187 = invoke class="VI" method="Default Vals.Reinit All"(reference=w56) -> ()  [unwired: 2 in, 3 out]
          n188 = property on="derivative time (Td, min)" class="DigNum (strict)"("NumText.Text"="0" ("Numeric Text.Text")) -> ()  [unwired: 2 in, 2 out]
        }
      }
      n189 = Unbundle By Name(w14) -> ("Settings.PID 2 Parameters.Input Device"=w15:enum16{"Default", "4-20mA"})
      n190 = case "Load settings if there are any written" shown="\"Bronkhorst M13\"..\"Scale Rate of Change\"" w15 {
        tunnel: w14 -> [_ w35]
        frame "Default", Default {
        }
        frame "Default", "4-20mA" {
          n191 = Unbundle By Name(w35) -> ("Settings"=w46:T3)
          n192 = Unbundle(w46) -> (w47:dbl, w48:T24, w36:dbl, w37:bool, w38:T4, w39:T5, w41, w43, w34, w33, w32, w31)  [unwired: 2 out]
          n193 = Unbundle(w39) -> (w44:refnum<k21>, w45, w40)  [unwired: 1 out]
          n194 = property on="Input Device" class="Enum (strict)"("Val(Sgnl)"=w44) -> ()  [unwired: 2 in, 2 out]
          n195 = property on="Output Device" class="Enum (strict)"("Val(Sgnl)"=w45) -> ()  [unwired: 2 in, 2 out]
          n196 = Bundle("Output DAQ Task"=w44, w45, w40) -> (w42:T25)  [unwired: 1 in]
          n197 = Bundle("Cycle Period"=w47, "PID 2 Parameters"=w48, "Manual Entry"=w36, "Auto?"=w37, "4-20mA Input Settings"=w38, w42, w41, w43, w34, w33, w32, w31) -> (w30:T26)  [unwired: 1 in]
          n198 = local write "Settings Dialog"(w30) -> ()
        }
      }
      n199 = disable-structure shown="Disabled" {
        disable-tunnel: w22 -> [w26 _]
        disable-tunnel: w17 -> [w25 _]
        frame Disabled {
          n200 = case shown="True" w25 {
            tunnel: w26 -> [_ w28]
            frame False {
            }
            frame True {
              # "Write settings back to XML"
              n201 = Flatten To XML(anything=w28) -> (xml string=w27:string)
              n202 = call "Get Config File Path.vi"() -> ("XML File Path"=w29:path)  [unwired: 10 in, 1 out]
              n203 = call-poly <vilib>:"Write to XML File.vi"("XML Input"=w27, "XML File Path"=w29) -> ()  [unwired: 7 in, 3 out]
            }
          }
        }
        frame Enabled {
        }
      }
    }
    frame Error {
    }
  }
  "UI Refresh Needed?" <- w10
  "error out" <- w11
  "Cancelled?" <- w9
  "PRM Config Out" <- w1
